vi "Average experiments.vi"(8 "error in (no error)":errorcluster, 9 "sigma":dbl, 10 "Name+Comments+bounds":T1, 11 "Control-Client in":refnum<class "Control-Client.lvclass">) -> (0 "error out":errorcluster, 3 "Control-Client out":refnum<class "Control-Client.lvclass">)   [LabVIEW 2015, in "Control-Client.lvclass"]
uses:
  Control-Client.lvclass
  Experiments/Experiment.lvclass
  Control-Client.lvclass/Control-Client.ctl
  Experiments/Experiment.lvclass/Experiment.ctl
  methods/Read Group #.vi
  Experiments/Experiments_group.lvclass
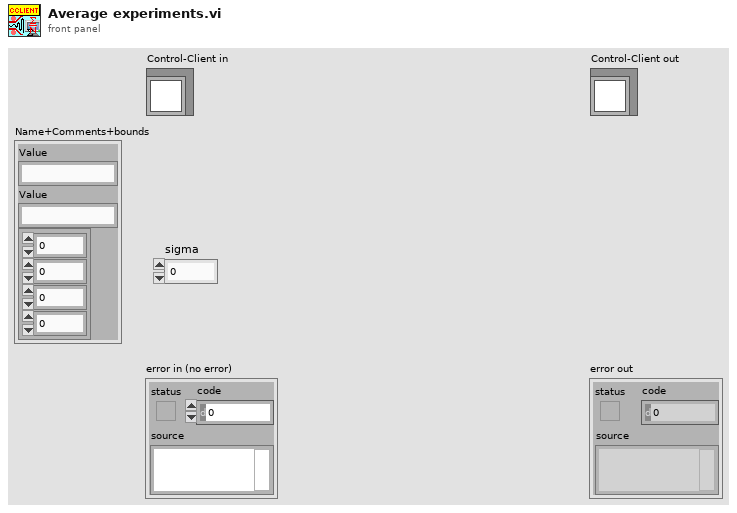
[diagram p1: front panel]
types:
  T1 = cluster{"Value":string, "Value":string, cluster{dbl, dbl, dbl, dbl}}
  T2 = typedef "mylistbox.ctl" = i32[]
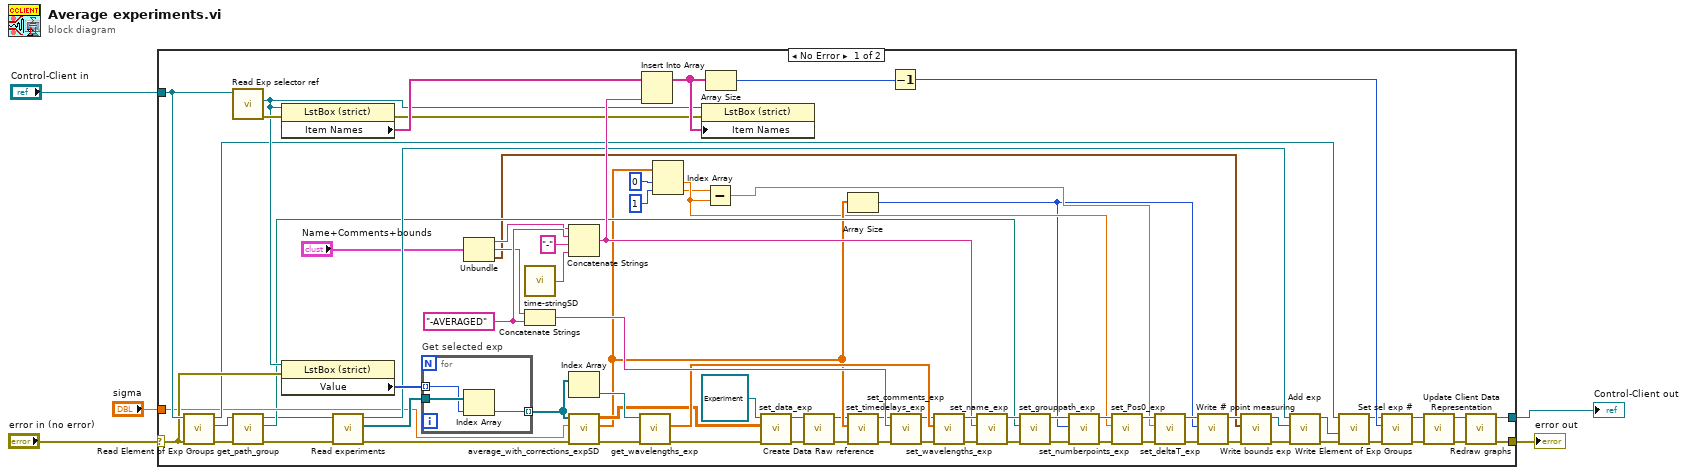
[diagram p0: block diagram]
diagram:
  n1 = case shown="No Error" "error in (no error)" {
    selector: "error in (no error)" -> [w53 w87]
    tunnel: [w42 w87] -> w4
    tunnel: [w41 w86] -> w2
    tunnel: "Control-Client in" -> [w54 w86]
    tunnel: "sigma" -> [w38 _]
    frame No Error {
      w77 = "-AVERAGED" ("string")
      n2 = call "Read Element of Exp Groups.vi"("error in (no error)"=w53, "Control-Client in"=w54) -> ("error out"=w35:errorcluster, "Experiments_group.lvclass"=w32:refnum<class "Experiments_group.lvclass">, "Control-Client out"=w50:refnum<class "Control-Client.lvclass">)  [unwired: 7 in]
      n3 = call "Read Exp selector ref.vi"("Control-Client in"=w54) -> ("error out"=w59:errorcluster, "Exp selector ref"=w57:refnum<vi>)  [unwired: 8 in, 1 out]
      n4 = call "get_path_group.vi"("error in (no error)"=w35, "Experiments_group.lvclass in"=w32) -> ("error out"=w34:errorcluster, "Path"=w33:path, "Experiments_group.lvclass out"=w31:refnum<class "Experiments_group.lvclass">)  [unwired: 7 in]
      n5 = property on="Property Node" class="LstBox (strict)"(reference=w57, error in=w59) -> (error out=w58:errorcluster, "Item Names"=w82:string[])  [unwired: 1 out]
      n6 = property class="LstBox (strict)"(reference=w57, error in=w53) -> ("Value"=w62:T2)  [unwired: 2 out]
      n7 = call "Read experiments.vi"("error in (no error)"=w34, "Experiments_group.lvclass in"=w31) -> ("error out"=w55:errorcluster, "Experiments"=w56:refnum<class "Experiment.lvclass">[], "Experiments_group.lvclass out"=w52:refnum<class "Experiments_group.lvclass">)  [unwired: 6 in]
      n8 = for "Get selected exp" {
        tunnel: w56 -> [w85]
        tunnel: w62 -> [w84] mode=indexing
        tunnel: [w83] -> w63 mode=indexing
        n9 = Index Array(array=w85, index=w84) -> (element=w83:refnum<class "Experiment.lvclass">)
      }
      n10 = Unbundle("Name+Comments+bounds") -> ("Value"=w76:string, "Value"=w73:string, w10:cluster{dbl, dbl, dbl, dbl})
      n11 = call "time-stringSD.vi"() -> ("time"=w75:string)
      n12 = Concatenate Strings(w73, w77) -> (w72:string)
      n13 = Concatenate Strings(w76, w77, "-" ("string"), w75) -> (w61:string)
      n14 = Index Array(array=w63) -> (element=w78:refnum<class "Experiment.lvclass">)  [unwired: 1 in]
      n15 = call "average_with_corrections_expSD.vi"("error in (no error)"=w55, "sigma"=w38, "all exp to average"=w63) -> ("sortie d'erreur"=w79:errorcluster, "timedelays longest"=w23:dbl[], "averaged without bad points"=w39:dbl[][])  [unwired: 6 in]
      n16 = call "get_wavelengths_exp.vi"("error in (no error)"=w79, "Experiment.lvclass in"=w78) -> ("error out"=w40:errorcluster, "wavelengths"=w71:dbl[])  [unwired: 7 in, 1 out]
      n17 = Insert Into Array(array=w82, new element=w61) -> (w81:string[])  [unwired: 1 in]
      n18 = Index Array(array=w23, index #1=0 ("index"), index #2=1 ("index")) -> (element #1=w20:dbl, element #2=w19:dbl)
      n19 = property on="Property Node" class="LstBox (strict)"(reference=w57, error in=w58, "Item Names"=w81) -> ()  [unwired: 2 out]
      n20 = Subtract(x=w19, y=w20) -> (x-y=w22:dbl)
      n21 = Array Size(array=w81) -> (size(s)=w80:i32)
      n22 = call "set_data_exp.vi"("error in (no error)"=w40, "Data"=w39, "Experiment.lvclass in"=refnum<class "Experiment.lvclass"> refnum) -> ("error out"=w6:errorcluster, "Experiment.lvclass out"=w9:refnum<class "Experiment.lvclass">)  [unwired: 7 in]
      n23 = call "Create Data Raw reference.vi"("error in (no error)"=w6, "Experiment in"=w9) -> ("error out"=w7:errorcluster, "Experiment out"=w8:refnum<class "Experiment.lvclass">)  [unwired: 8 in]
      n24 = Array Size(array=w23) -> (size(s)=w16:i32)
      n25 = call "set_timedelays_exp.vi"("error in (no error)"=w7, "timedelays"=w23, "Experiment.lvclass in"=w8) -> ("error out"=w68:errorcluster, "Experiment.lvclass out"=w65:refnum<class "Experiment.lvclass">)  [unwired: 7 in]
      n26 = Decrement(x=w80) -> (x-1=w60:i32)
      n27 = call "set_comments_exp.vi"("error in (no error)"=w68, "Comments"=w72, "Experiment.lvclass in"=w65) -> ("error out"=w69:errorcluster, "Experiment.lvclass out"=w66:refnum<class "Experiment.lvclass">)  [unwired: 7 in]
      n28 = call "set_wavelengths_exp.vi"("error in (no error)"=w69, "wavelengths"=w71, "Experiment.lvclass in"=w66) -> ("error out"=w70:errorcluster, "Experiment.lvclass out"=w67:refnum<class "Experiment.lvclass">)  [unwired: 7 in]
      n29 = call "set_name_exp.vi"("error in (no error)"=w70, "Exp name"=w61, "Experiment.lvclass in"=w67) -> ("error out"=w37:errorcluster, "Experiment.lvclass out"=w36:refnum<class "Experiment.lvclass">)  [unwired: 7 in]
      n30 = call "set_grouppath_exp.vi"("error in (no error)"=w37, "GroupPath"=w33, "Experiment.lvclass in"=w36) -> ("error out"=w27:errorcluster, "Experiment.lvclass out"=w28:refnum<class "Experiment.lvclass">)  [unwired: 7 in]
      n31 = call "set_numberpoints_exp.vi"("error in (no error)"=w27, "numberpoints"=w16, "Experiment.lvclass in"=w28) -> ("error out"=w26:errorcluster, "Experiment.lvclass out"=w30:refnum<class "Experiment.lvclass">)  [unwired: 6 in]
      n32 = call "set_Pos0_exp.vi"("error in (no error)"=w26, "Pos0,ps"=w20, "Experiment.lvclass in"=w30) -> ("error out"=w25:errorcluster, "Experiment.lvclass out"=w29:refnum<class "Experiment.lvclass">)  [unwired: 6 in]
      n33 = call "set_deltaT_exp.vi"("error in (no error)"=w25, "deltaTlast"=w22, "Experiment.lvclass in"=w29) -> ("error out"=w17:errorcluster, "Experiment.lvclass out"=w18:refnum<class "Experiment.lvclass">)  [unwired: 6 in]
      n34 = call "Write # point measuring.vi"("error in (no error)"=w17, "# point measuring"=w16, "Experiment in"=w18) -> ("error out"=w14:errorcluster, "Experiment out"=w11:refnum<class "Experiment.lvclass">)  [unwired: 7 in]
      n35 = call "Write bounds exp.vi"("error in (no error)"=w14, "Bounds"=w10, "Experiment in"=w11) -> ("error out"=w13:errorcluster, "Experiment out"=w12:refnum<class "Experiment.lvclass">)  [unwired: 7 in]
      n36 = call "Add exp.vi"("error in (no error)"=w13, "New exp"=w12, "Experiments_group in"=w52) -> ("error out"=w47:errorcluster, "Experiments_group out"=w51:refnum<class "Experiments_group.lvclass">)  [unwired: 7 in]
      n37 = call "Write Element of Exp Groups.vi"("error in (no error)"=w47, "Experiments_group.lvclass"=w51, "Control-Client in"=w50) -> ("error out"=w48:errorcluster, "Control-Client out"=w49:refnum<class "Control-Client.lvclass">)  [unwired: 7 in]
      n38 = call "Set sel exp #.vi"("error in (no error)"=w48, "Exp sel #"=w60, "Control-Client in"=w49) -> ("error out"=w45:errorcluster, "Control-Client out"=w46:refnum<class "Control-Client.lvclass">)  [unwired: 7 in]
      n39 = call "Update Client Data Representation.vi"("error in (no error)"=w45, "Control-Client in"=w46) -> ("error out"=w44:errorcluster, "Control-Client out"=w43:refnum<class "Control-Client.lvclass">)  [unwired: 8 in]
      n40 = call "Redraw graphs.vi"("error in (no error)"=w44, "Control-Client in"=w43) -> ("error out"=w42:errorcluster, "Control-Client out"=w41:refnum<class "Control-Client.lvclass">)  [unwired: 8 in]
    }
    frame Error {
    }
  }
  "error out" <- w4
  "Control-Client out" <- w2
